vi "PLC.ReadDataBlock.vi"(8 "error in (no error)":errorcluster, 9 "Amount (1)":i32=1, 10 "Block":i32, 11 "Ref":u64) -> (0 "error out":errorcluster, 2 "data out":u8[](array[numeric]) format="%02x", 3 "ref out":u64)   [LabVIEW 2016]
doc: "ReadDataBlock\n\nWabco 2017 All right reserved\nAuthor: maciej.szupienko@wabco-auto.com"
uses:
  Snap7/lib/Snap7.lvlib
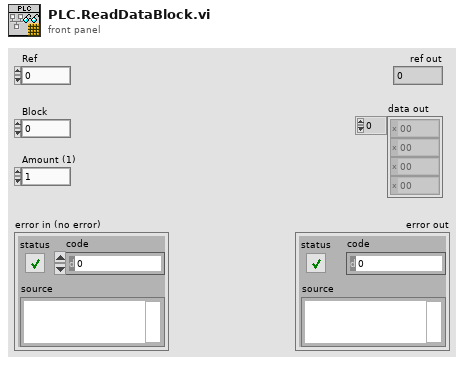
[diagram p1: front panel]
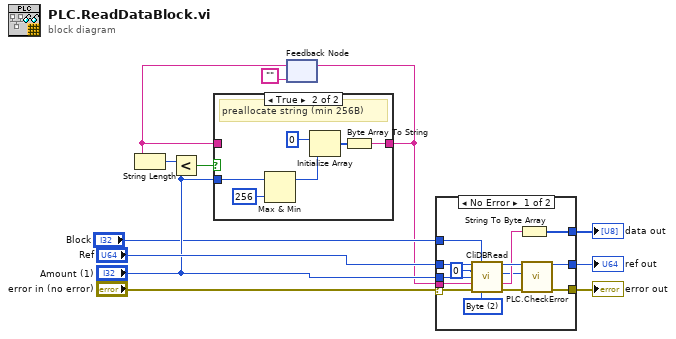
[diagram p0: block diagram]
diagram:
  n1 = feedback #1("") -> (w8:string)
  n2 = String Length(string=w8) -> (length=w6:i32)
  n3 = Less?(x=w6, y="Amount (1)") -> (x < y?=w5:bool)
  n4 = case shown="True" w5 {
    tunnel: [w13 w16] -> w1
    tunnel: w8 -> [w13 _]
    tunnel: "Amount (1)" -> [_ w15]
    frame False {
    }
    frame True {
      # "preallocate string (min 256B)"
      n5 = Max & Min(x=w15, y=256) -> (max(x,y)=w14:i32)  [unwired: 1 out]
      n6 = Initialize Array(u8 0, w14) -> (w17:u8[])
      n7 = Byte Array To String(unsigned byte array=w17) -> (string=w16:string)
    }
  }
  n8 = feedback-in #1(w1) -> ()
  n9 = case shown="No Error" "error in (no error)" {
    selector: "error in (no error)" -> [w27 w34]
    tunnel: [w22 w34] -> w12
    tunnel: [w32 w33] -> w11
    tunnel: w1 -> [w30 _]
    tunnel: "Amount (1)" -> [w29 _]
    tunnel: "Ref" -> [w28 w33]
    tunnel: [w25 _] -> w3
    tunnel: "Block" -> [w21 _]
    frame No Error {
      w31 = 2 items=["Bit"=1, "Byte"=2, "Word"=4, "DWord"=6, "Real"=8, "Counter"=28, "Timer"=29] ("Word Length")
      n10 = call "CliDBRead.vi"("ref in"=w28, "DB Number"=w21, "Start"=0 ("DB Number"), "Amount"=w29, "data in"=w30, "error in (no error)"=w27, "Word Length"=w31) -> ("ref out"=w32:u64, "Result"=w23:i32, "data out"=w26:string, "error out"=w24:errorcluster)  [unwired: 5 in]
      n11 = String To Byte Array(string=w26) -> (unsigned byte array=w25:u8[])
      n12 = call "PLC.CheckError.vi"("error in (no error)"=w24, "Result"=w23) -> ("error out"=w22:errorcluster)  [unwired: 9 in]
    }
    frame Error {
    }
  }
  "error out" <- w12
  "ref out" <- w11
  "data out" <- w3
